vi "demo_G2CPU GPU Toolkit.vi"(11 "Stop Demo":refnum<user-event>) -> ()   [LabVIEW 2020]
panel:
  # "The most complete GPU library for LabVIEW - Over 20GByte/s transfer and process rate\n\nNo more creating code that will run on only one platform. Create you algorithm in G²CPU and let the backend do the rest. Running it on a CUDA enabled device, an OpenCL GPU or fall back to the CPU whilst enabling multithreading. Now with Multi-GPU support and ability to run on LabVIEW RT targets\nhttps://g2cpu.com/"
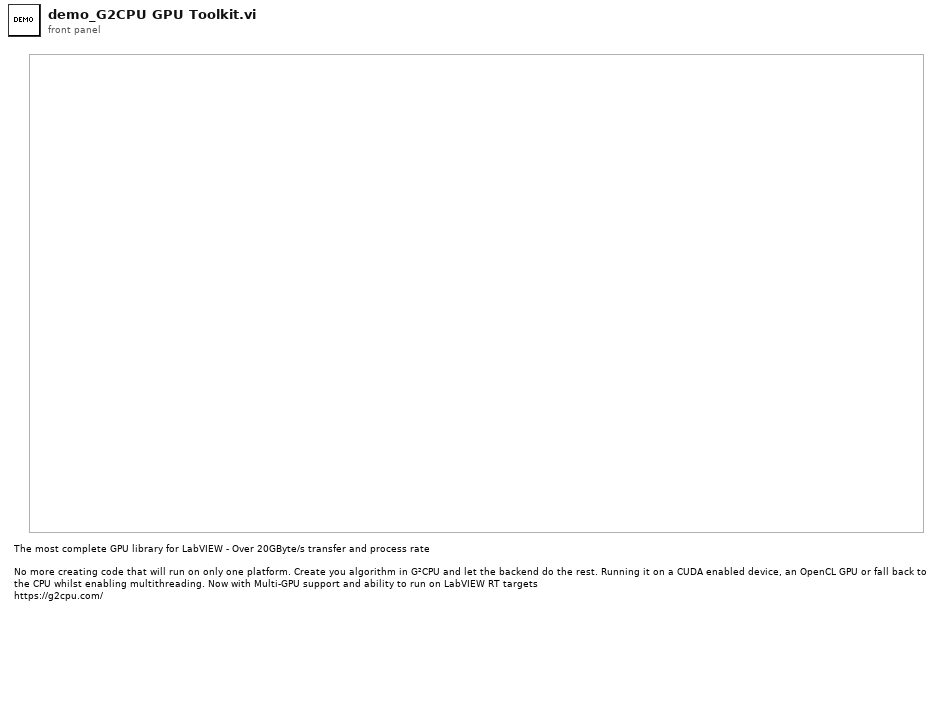
[diagram p1: front panel]
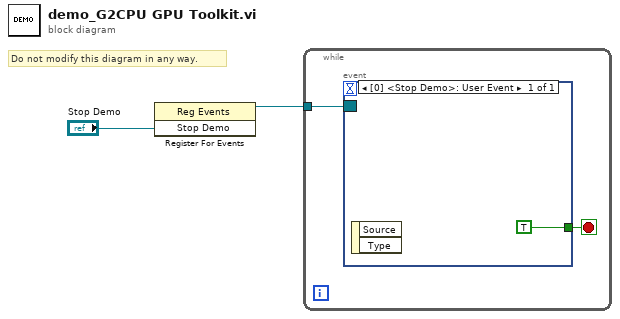
[diagram p0: block diagram]
diagram:
  # "Do not modify this diagram in any way."
  n1 = register-events("Stop Demo") -> (reference out=w1:refnum<event-registration>)  [unwired: 2 in, 1 out]
  n2 = while {
    tunnel: w1 -> [w4]
    stop <- w3 stop-if-true
    n3 = event shown="[0] <Stop Demo>: User Event" {
      selector: w4 -> [_]
      dyn-events: _ -> [_]
      timeout: _ -> [_]
      tunnel: [TRUE] -> w3
      event User Event {
        n4 = event-data() -> ()  [unwired: 1 in, 2 out]
      }
    }
  }
